vi "ShowBinary.vi"() -> ()   [LabVIEW 2015]
panel:
  in  "stop":bool
  out "Numeric in binary":u16 format="%0.0f"
  out "resulting string":string
  in  "Numeric":u16 format="%16b"
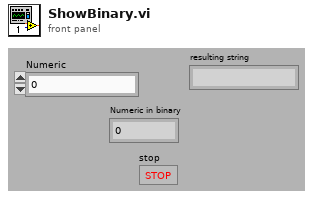
[diagram p1: front panel]
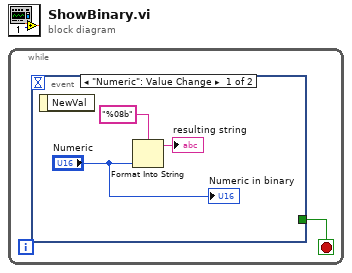
[diagram p0: block diagram]
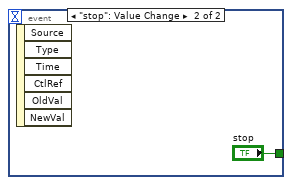
[diagram p2: hidden frame]
diagram:
  n1 = while {
    stop <- w1 stop-if-true
    n2 = event shown="[0] \"Numeric\": Value Change" {
      selector: _ -> [_ _]
      dyn-events: _ -> [_ _]
      timeout: _ -> [_ _]
      tunnel: [_ "stop"] -> w1
      event "Numeric": Value Change {
        n3 = event-data() -> ()  [unwired: 1 in, 1 out]
        n4 = Format Into String(format string="%08b", "Numeric") -> (resulting string=→"resulting string":string)  [unwired: 2 in, 1 out]
        "Numeric in binary" <- "Numeric"
      }
      event "stop": Value Change {
        n5 = event-data() -> ()  [unwired: 1 in, 6 out]
      }
    }
  }
